vi "GetFunctionSampleRate.vi"(8 "error in (no error)":errorcluster, 11 "ArbitraryFunction in":refnum<class "ArbitraryFunction.lvclass">) -> (0 "error out":errorcluster, 2 "SampleRate":variant, 3 "ArbitraryFunction out":refnum<class "ArbitraryFunction.lvclass">)   [LabVIEW 2018, in "Functions.lvlib" / "ArbitraryFunction.lvclass"]
uses:
  ArbitraryFunction.lvclass
  ArbitraryFunction.lvclass/ArbitraryFunction.ctl
  Accessors/Read SampleRate.vi
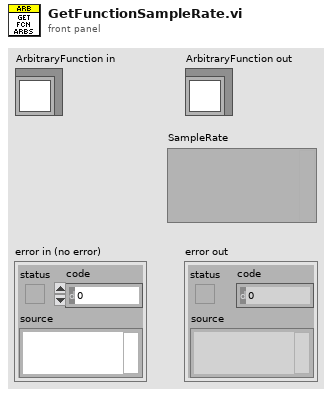
[diagram p1: front panel]
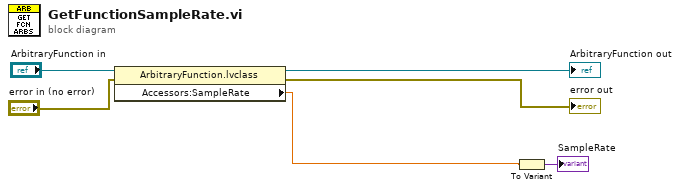
[diagram p0: block diagram]
diagram:
  n1 = property class="ArbitraryFunction.lvclass"(reference="ArbitraryFunction in", error in="error in (no error)") -> (reference out=→"ArbitraryFunction out":refnum<class "ArbitraryFunction.lvclass">, error out=→"error out":errorcluster, "Accessors:SampleRate"=w1:dbl)
  n2 = To Variant(anything=w1) -> (Variant=→"SampleRate":variant)
